vi "RotateY.vi"(8 "error in (no error)":errorcluster, 9 "radians":dbl, 10 "Modelview in":dbl[][](array[numeric])=[[1.0, 0.0, 0.0, 0.0], [0.0, 1.0, 0.0, 0.0], [0.0, 0.0, 1.0, 0.0], [0.0, 0.0, 0.0, 1.0]], 11 "3D Scene in":refnum<class "3D Scene.lvclass">) -> (0 "error out":errorcluster, 2 "Modelview out":dbl[][](array[numeric]), 3 "3D Scene out":refnum<class "3D Scene.lvclass">)   [LabVIEW 2015, in "3D Scene.lvclass"]
uses:
  3D Scene.lvclass
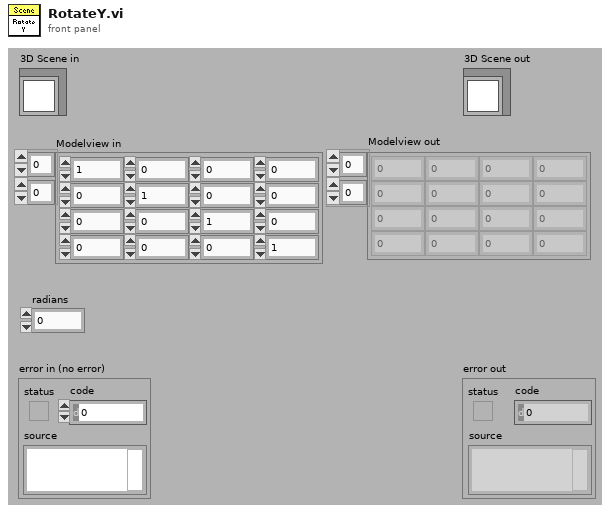
[diagram p1: front panel]
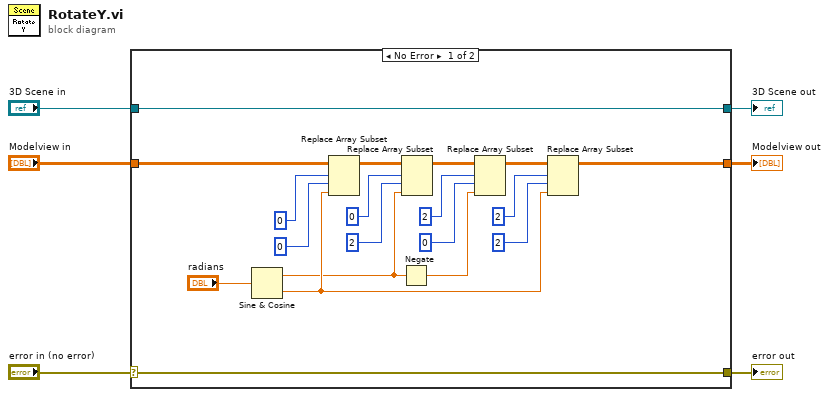
[diagram p0: block diagram]
diagram:
  n1 = case shown="No Error" "error in (no error)" {
    selector: "error in (no error)" -> [w24 w28]
    tunnel: [w24 w28] -> w5
    tunnel: [w25 w27] -> w3
    tunnel: "3D Scene in" -> [w25 w27]
    tunnel: "Modelview in" -> [w8 w26]
    tunnel: [w7 w26] -> w1
    frame No Error {
      n2 = Sine & Cosine(0:"radians") -> (1:w20:dbl, 2:w22:dbl)
      n3 = Replace Array Subset(array=w8, new element=w22, index (row)=0, index (col)=0 ("disabled index (col)")) -> (w9:dbl[][])
      n4 = Negate(x=w20) -> (-x=w21:dbl)
      n5 = Replace Array Subset(array=w9, new element=w20, index (row)=0 ("disabled index (row)"), index (col)=2 ("disabled index (col)")) -> (w10:dbl[][])
      n6 = Replace Array Subset(array=w10, new element=w21, index (row)=2, index (col)=0 ("disabled index (col)")) -> (w11:dbl[][])
      n7 = Replace Array Subset(array=w11, new element=w22, index (row)=2, index (col)=2 ("disabled index (col)")) -> (w7:dbl[][])
    }
    frame Error {
    }
  }
  "error out" <- w5
  "3D Scene out" <- w3
  "Modelview out" <- w1
